vi "I2C_WriteQuick.vi"(5 "Bus":i32=1, 7 "Address":u8 format="%.0x", 8 "error in":errorcluster) -> (0 "error out":errorcluster)   [LabVIEW 2014]
doc: "Sends a single bit to the device"
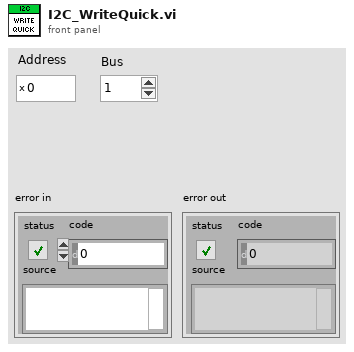
[diagram p1: front panel]
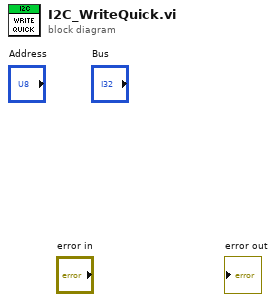
[diagram p0: block diagram]
diagram:
